vi "Send Template.vi"(7 "Message Priority (Normal)":T1=enum."Normal", 8 "error in (no error)":errorcluster, 11 "send queue":refnum<class "Send Queue.lvclass">) -> (0 "error out":errorcluster)   [LabVIEW 2011, in "Message Template.lvclass"]
uses:
  Message Template.lvclass
  <vilib>/ActorFramework/Send Queue/Send Queue.lvclass
  <vilib>/ActorFramework/Send Queue/Message Priority.ctl
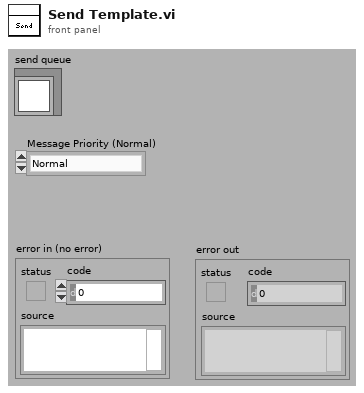
[diagram p1: front panel]
types:
  T1 = typedef "Actor Framework.lvlib/Send Queue.lvclass/Message Priority.ctl" = enum16{"Low", "Normal", "High"}
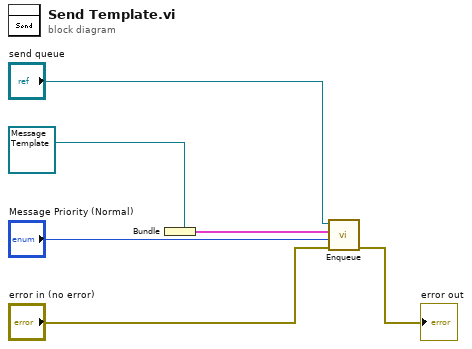
[diagram p0: block diagram]
diagram:
  n1 = Bundle(cluster=refnum<class "Message Template.lvclass"> refnum ("Object")) -> (w2:cluster{void})  [unwired: 1 in]
  n2 = call <vilib>:"Enqueue.vi"("error in (no error)"="error in (no error)", "Message Priority (Normal)"="Message Priority (Normal)", "Message"=w2, "Send Queue in"="send queue") -> ("error out"=→"error out":errorcluster)  [unwired: 6 in, 1 out]
